vi "start.vi"(8 "error in (no error)":errorcluster, 11 "DL090211DAQScaffold in":refnum<class "DAQ_DL090211Scaffold.lvclass">) -> (0 "error out":errorcluster, 3 "DL090211DAQScaffold out":refnum<class "DAQ_DL090211Scaffold.lvclass">)   [LabVIEW 2010, in "DAQ_DL090211Scaffold.lvclass"]
uses:
  DAQ_DL090211Scaffold.lvclass
  GenericDAQ/GenericDAQ/GenericDAQ.lvclass
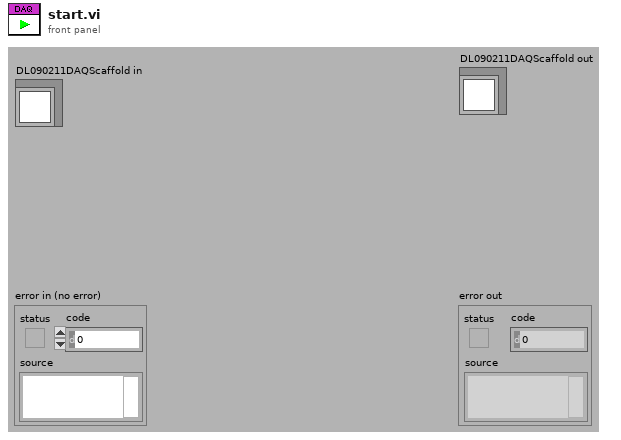
[diagram p1: front panel]
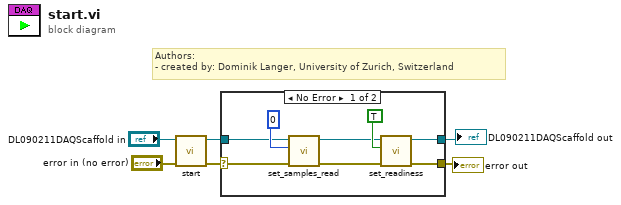
[diagram p0: block diagram]
diagram:
  # "Authors: \n- created by: Dominik Langer, University of Zurich, Switzerland"
  n1 = call-parent "start.vi"("error in (no error)"="error in (no error)", "GenericToplevelComponent in"="DL090211DAQScaffold in") -> ("error out"=w1:errorcluster, "GenericToplevelComponent out"=w3:refnum<class "DAQ_DL090211Scaffold.lvclass">)  [unwired: 8 in]
  n2 = case shown="No Error" w1 {
    selector: w1 -> [w13 w16]
    tunnel: [w9 w16] -> w6
    tunnel: [w7 w15] -> w5
    tunnel: w3 -> [w12 w15]
    frame No Error {
      n3 = call-dynamic "set_samples_read.vi"("error in (no error)"=w13, "samples read"=i64 0 ("pixels read"), "GenericDAQ.lvclass in"=w12) -> ("error out"=w10:errorcluster, "GenericDAQ.lvclass out"=w8:refnum<class "DAQ_DL090211Scaffold.lvclass">)  [unwired: 7 out]
      n4 = call-dynamic "set_readiness.vi"("error in (no error)"=w10, "ready?"=TRUE, "DAQ_DL090211Scaffold in"=w8) -> ("error out"=w9:errorcluster, "DAQ_DL090211Scaffold out"=w7:refnum<class "DAQ_DL090211Scaffold.lvclass">)  [unwired: 7 in]
    }
    frame Error {
    }
  }
  "error out" <- w6
  "DL090211DAQScaffold out" <- w5
